vi "Append to Data (Dictionary).vi"(8 "error in (no error)":errorcluster, 10 "key-value":cluster{"key":string, "value":variant}, 11 "Data Save":refnum<class "Data.lvclass">) -> (0 "error out":errorcluster, 3 "Data Save out":refnum<class "Data.lvclass">)   [LabVIEW 2016, in "Data.lvclass"]
uses:
  Data.lvclass
  Data.lvclass/Data.ctl
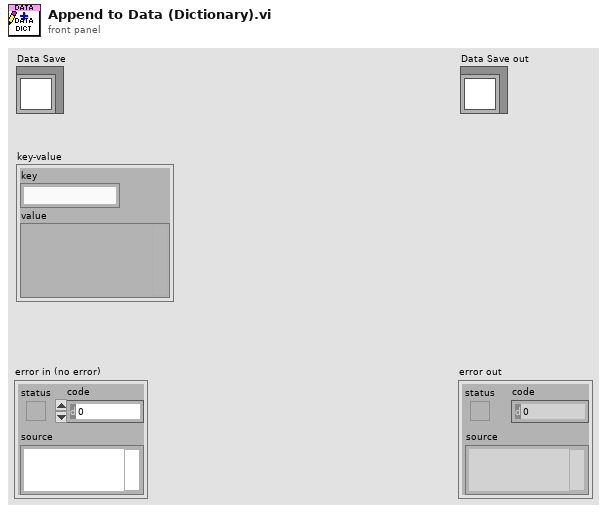
[diagram p1: front panel]
types:
  T1 = typedef "Data.lvclass/Dictionary--cluster.ctl" = cluster{"key":string, "value":variant}
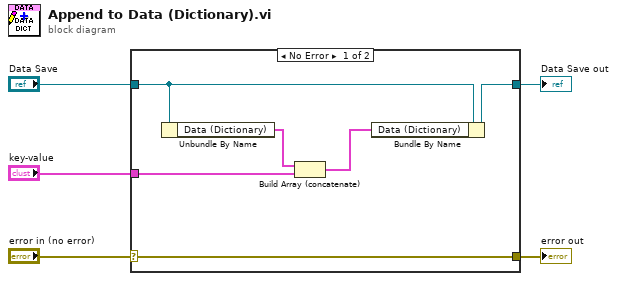
[diagram p0: block diagram]
diagram:
  n1 = case shown="No Error" "error in (no error)" {
    selector: "error in (no error)" -> [w11 w12]
    tunnel: [w11 w12] -> w4
    tunnel: [w10 w13] -> w2
    tunnel: "Data Save" -> [w9 w13]
    tunnel: "key-value" -> [w7 _]
    frame No Error {
      n2 = Unbundle By Name(w9) -> ("Data (Dictionary)"=w8:T1[])
      n3 = Build Array (concatenate)(w8, w7) -> (w6:T1[])
      n4 = Bundle By Name(cluster=w9, "Data (Dictionary)"=w6) -> (w10:refnum<class "Data.lvclass">)
    }
    frame Error {
    }
  }
  "error out" <- w4
  "Data Save out" <- w2
